vi "ArrayFile.vi"(11 "File Path":string) -> (3 "Error out":errorcluster, 8 "Array":dbl[](array[numeric]))   [LabVIEW 2014]
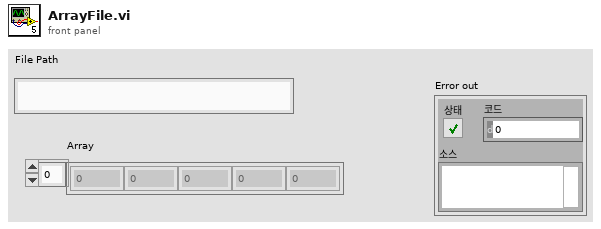
[diagram p1: front panel]
types:
  T1 = enum16{"open", "replace", "create", "open or create", "replace or create", "replace or create with confirmation"}
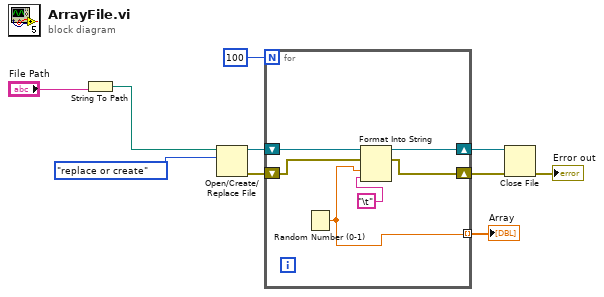
[diagram p0: block diagram]
diagram:
  n1 = String To Path(string="File Path") -> (path=w5:path)
  n2 = Open/Create/Replace File(file path (use dialog)=w5, operation (0:open)=T1."replace or create" ("동작(0:open)")) -> (refnum out=w10:refnum<file>, error out=w9:errorcluster)  [unwired: 4 in, 1 out]
  n3 = for {
    N: 100 -> [_]
    shift-right: [w14] -> w8
    shift-left: w10 -> [w16]
    shift-right: [w13] -> w7
    shift-left: w9 -> [w15]
    tunnel: [w12] -> w2 mode=indexing
    n4 = Random Number (0-1)() -> (number: 0 to 1=w12:dbl)
    n5 = Format Into String(initial string=w16, error in=w15, w12, "\t") -> (resulting string=w14:refnum<file>, error out=w13:errorcluster)  [unwired: 1 in]
  }
  "Array" <- w2
  n6 = Close File(refnum=w8, error in=w7) -> (error out=→"Error out":errorcluster)  [unwired: 1 out]
